vi "Set Path Values.vi"(7 "Target (Process)":T1 items=["Process", "User", "Machine"], 8 "Error In":errorcluster, 11 "Values[]":string[](array[string])) -> (0 "Error Out":errorcluster)   [LabVIEW 2023, in "SLL Environment Variable.lvlib"]
doc: "Set the <B>Values[]</B> to path variable in the target environment."
uses:
  SLL Environment Variable.lvlib
  _Typedef/Target Environment Enum.ctl
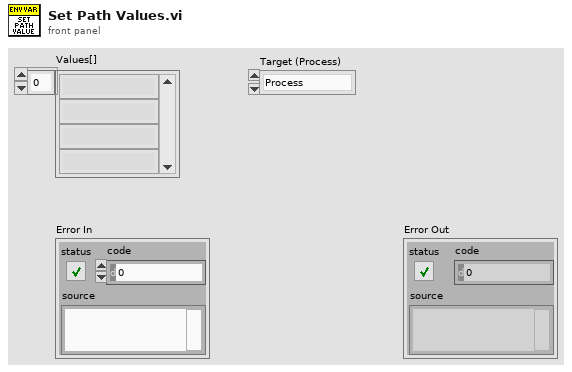
[diagram p1: front panel]
types:
  T1 = typedef "SLL Environment Variable.lvlib/Target Environment Enum.ctl" = i32
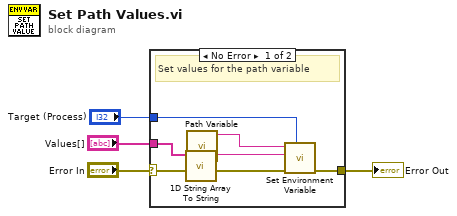
[diagram p0: block diagram]
diagram:
  n1 = case shown="No Error" "Error In" {
    selector: "Error In" -> [w5 w11]
    tunnel: [w9 w11] -> w4
    tunnel: "Target (Process)" -> [w8 _]
    tunnel: "Values[]" -> [w7 _]
    frame No Error {
      # "Set values for the path variable"
      n2 = call "1D String Array To String.vi"("Array[]"=w7) -> ("String"=w10:string)  [unwired: 10 in]
      n3 = call "Path Variable.vi"() -> ("Path Variable"=w6:string)  [unwired: 11 in]
      n4 = call "Set Environment Variable.vi"("Target (Process)"=w8, "Error In"=w5, "Value"=w10, "Name"=w6) -> ("Error Out"=w9:errorcluster)  [unwired: 7 in]
    }
    frame Error {
    }
  }
  "Error Out" <- w4
